vi "Test Power Spectrum.vi"(2 "Power Spectrum In":dynamicdata(graph), 3 "Signal In":dynamicdata(graph)) -> (0 "error out":errorcluster, 1 "Equal":bool)   [LabVIEW 2010]
uses:
  <vilib>/express/express analysis/Spectral/XNode/ExpressSpectralMeasurementsBlockNode.xnode
  Instance           2 27Saved   Test Power Spectrum .vi
  <vilib>/express/express analysis/Spectral/Block/exnSpectralBlock spectral measurements power poly.vi
  <vilib>/express/express analysis/Spectral/Block/exnSpectralBlock spectral measurements power DDT.vi
panel:
  out "Power Spectrum":dynamicdata(graph)
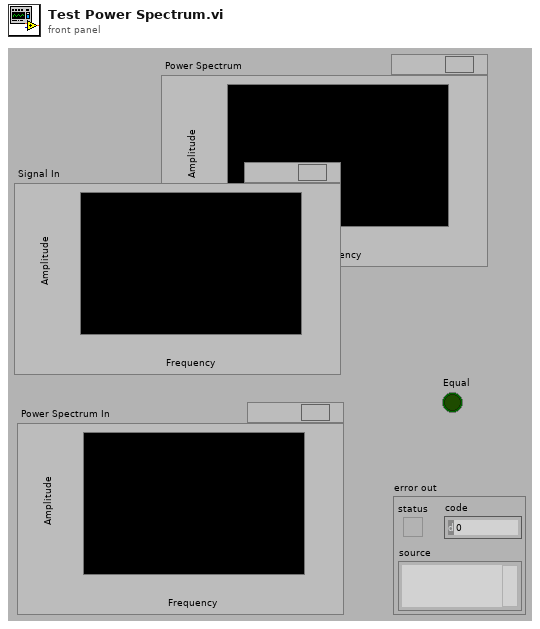
[diagram p1: front panel]
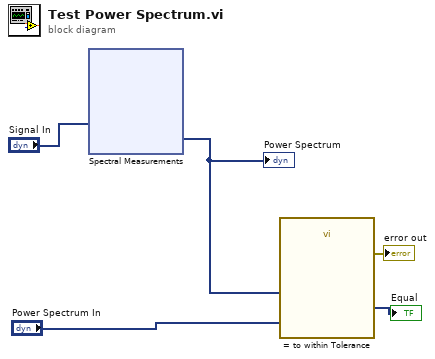
[diagram p0: block diagram]
diagram:
  n1 = xnode "Spectral Measurements"("Signals"="Signal In") -> ("Power Spectrum"=w2:dynamicdata)  [unwired: 1 in, 1 out]
  "Power Spectrum" <- w2
  n2 = call "= to within Tolerance"("Operand 2"="Power Spectrum In", "Operand 1"=w2) -> ("error out"=→"error out":errorcluster, "Result"=→"Equal":dynamicdata)  [unwired: 1 in, 7 out]
